vi "Modify Task ID and Name in Map.vi"(4 "List In":refnum<vi>, 6 "New Name":string, 8 "error in (no error)":errorcluster, 9 "New ID":i64, 10 "Original ID":i64, 11 "Composite Map Task in":refnum<class "Composite ID-Map Task.lvclass">) -> (0 "error out":errorcluster, 3 "Composite Map Task out":refnum<class "Composite ID-Map Task.lvclass">)   [LabVIEW 2024, in "Composite ID-Map Task.lvclass"]
uses:
  Composite ID-Map Task.lvclass
  Composite ID-Map Task.lvclass/Composite ID-Map Task.ctl
  Task Ancestor/Task Ancestor.lvclass/Task Ancestor.ctl
  Task Ancestor/Public Data/Write Task Name.vi
  Public Data/Read Task Map.vi
  Public Data/Write Task Map.vi
  Polymorphic VIs/Reference Manipulation/List/List-Modify Item Name(Keep ID).vi
  Polymorphic VIs/Reference Manipulation/List/List-Remove Current Item.vi
  Polymorphic VIs/Reference Manipulation/List/List-Item Name From ID and Name .vi
  Polymorphic VIs/Reference Manipulation/List/List-Sort Item Names.vi
  Task Ancestor/Task Ancestor.lvclass
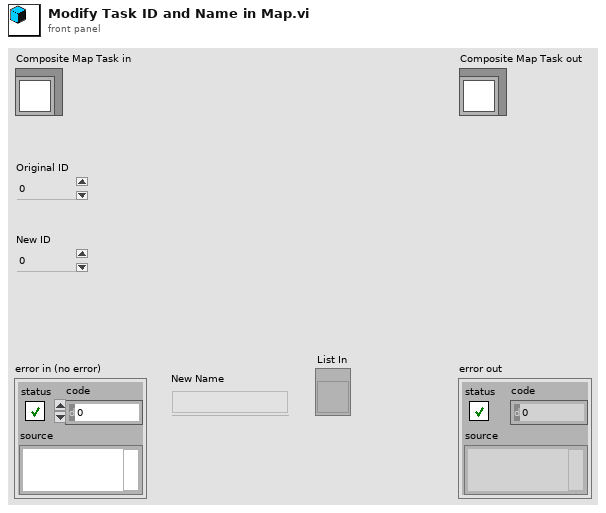
[diagram p1: front panel]
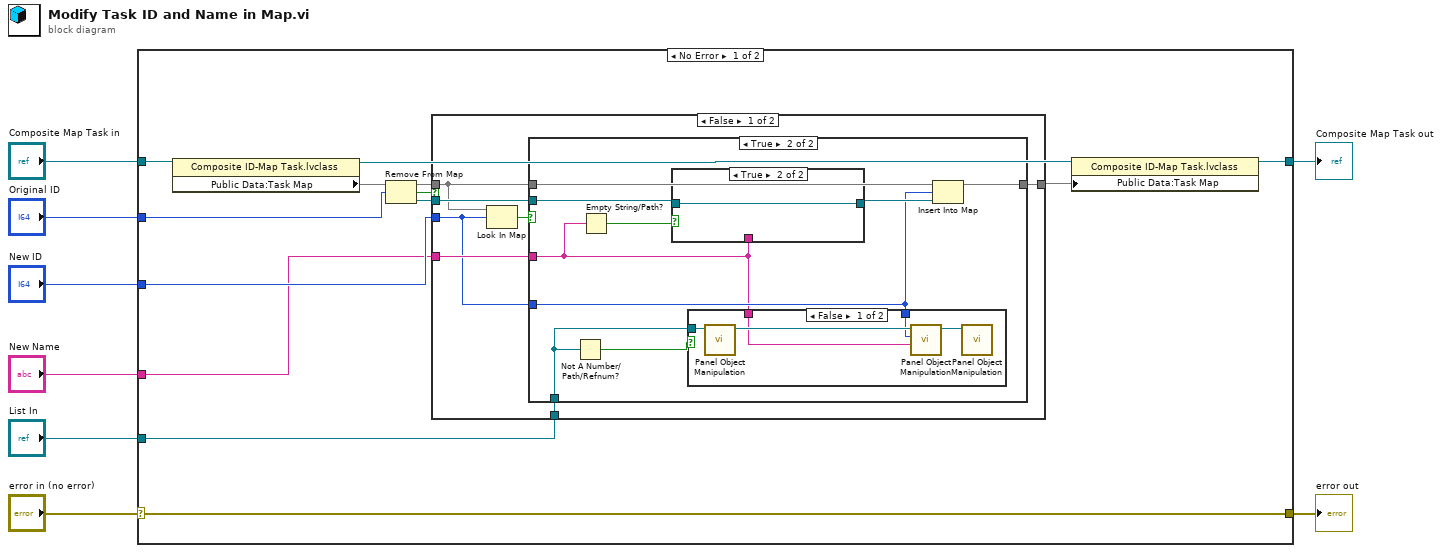
[diagram p0: block diagram]
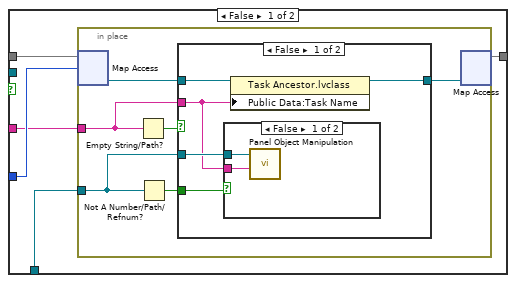
[diagram p2: hidden frame]
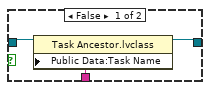
[diagram p5: hidden frame]
diagram:
  n1 = case shown="No Error" "error in (no error)" {
    selector: "error in (no error)" -> [w21 w68]
    tunnel: [w21 w68] -> w7
    tunnel: [w13 w67] -> w5
    tunnel: "Composite Map Task in" -> [w14 w67]
    tunnel: "Original ID" -> [w12 _]
    tunnel: "New ID" -> [w11 _]
    tunnel: "New Name" -> [w10 _]
    tunnel: "List In" -> [w9 _]
    frame No Error {
      n2 = property class="Composite ID-Map Task.lvclass"(reference=w14) -> (reference out=w20:refnum<class "Composite ID-Map Task.lvclass">, "Public Data:Task Map"=w19:map{i64, refnum<class "Task Ancestor.lvclass">})  [unwired: 1 in, 1 out]
      n3 = Remove From Map(10:w12, 11:w19) -> (1:w15:refnum<class "Task Ancestor.lvclass">, 2:w18:bool, 3:w17:map{i64, refnum<class "Task Ancestor.lvclass">})
      n4 = case shown="False" w18 {
        tunnel: w17 -> [w25 w66]
        tunnel: [w26 w66] -> w16
        tunnel: w15 -> [w28 _]
        tunnel: w10 -> [w27 _]
        tunnel: w11 -> [w22 _]
        tunnel: w9 -> [w23 _]
        frame False {
          n5 = Look In Map(map=w25, key=w22) -> (key not found?=w24:bool)  [unwired: 1 in, 1 out]
          n6 = case shown="True" w24 {
            tunnel: w28 -> [_ w56]
            tunnel: w27 -> [w30 w48]
            tunnel: [w32 w54] -> w26
            tunnel: w25 -> [w33 w53]
            tunnel: w23 -> [w29 w51]
            tunnel: w22 -> [w31 w52]
            frame False {
              n7 = in-place {
                in-place-border: w30 -> [w36]
                in-place-border: w29 -> [w34]
                n8 = in-place-map #1(w33, w31) -> (w38:refnum<class "Task Ancestor.lvclass">)  [unwired: 1 in, 1 out]
                n9 = Empty String/Path?(string/path=w36) -> (empty?=w39:bool)
                n10 = Not A Number/Path/Refnum?(number/path/refnum=w34) -> (NaN/Path/Refnum?=w35:bool)
                n11 = case shown="False" w39 {
                  tunnel: [w44 w47] -> w37
                  tunnel: w38 -> [w43 w47]
                  tunnel: w36 -> [w40 _]
                  tunnel: w35 -> [w42 _]
                  tunnel: w34 -> [w41 _]
                  frame False {
                    n12 = case shown="False" w42 {
                      tunnel: w41 -> [w46 _]
                      tunnel: w40 -> [w45 _]
                      frame False {
                        n13 = call-poly "Panel Object Manipulation.vi"("New Name"=w45, "List in"=w46) -> ()  [unwired: 9 in, 1 out]
                      }
                      frame True {
                      }
                    }
                    n14 = property class="Task Ancestor.lvclass"(reference=w43, "Public Data:Task Name"=w40) -> (reference out=w44:refnum<class "Task Ancestor.lvclass">)  [unwired: 1 in, 1 out]
                  }
                  frame True {
                  }
                }
                n15 = in-place-map #1(w37) -> (w32:map{i64, refnum<class "Task Ancestor.lvclass">})  [unwired: 1 in, 2 out]
              }
            }
            frame True {
              n16 = Not A Number/Path/Refnum?(number/path/refnum=w51) -> (NaN/Path/Refnum?=w50:bool)
              n17 = Empty String/Path?(string/path=w48) -> (empty?=w49:bool)
              n18 = case shown="True" w49 {
                tunnel: w56 -> [w59 w60]
                tunnel: [w58 w60] -> w55
                tunnel: w48 -> [w57 _]
                frame False {
                  n19 = property class="Task Ancestor.lvclass"(reference=w59, "Public Data:Task Name"=w57) -> (reference out=w58:refnum<class "Task Ancestor.lvclass">)  [unwired: 1 in, 1 out]
                }
                frame True {
                }
              }
              n20 = case shown="False" w50 {
                tunnel: w48 -> [w64 _]
                tunnel: w52 -> [w63 _]
                tunnel: w51 -> [w62 _]
                frame False {
                  n21 = call-poly "Panel Object Manipulation.vi"("List in"=w62) -> ("List Out"=w65:refnum<vi>)  [unwired: 10 in]
                  n22 = call-poly "Panel Object Manipulation.vi"("Name"=w64, "ID"=w63, "List"=w65) -> ("List Out"=w61:refnum<vi>)  [unwired: 8 in]
                  n23 = call-poly "Panel Object Manipulation.vi"("List in"=w61) -> ()  [unwired: 10 in, 1 out]
                }
                frame True {
                }
              }
              n24 = Insert Into Map(map in=w53, key=w52, value=w55) -> (map out=w54:map{i64, refnum<class "Task Ancestor.lvclass">})  [unwired: 2 out]
            }
          }
        }
        frame True {
        }
      }
      n25 = property class="Composite ID-Map Task.lvclass"(reference=w20, "Public Data:Task Map"=w16) -> (reference out=w13:refnum<class "Composite ID-Map Task.lvclass">)  [unwired: 1 in, 1 out]
    }
    frame Error {
    }
  }
  "error out" <- w7
  "Composite Map Task out" <- w5
